vi "writeToXMLAzimuth.vi"(8 "error in (no error)":errorcluster, 10 "Class Label":string="Azimuth") -> (0 "error out":errorcluster, 2 "XML out":string="<Azimuth>\n  <degreesArc>0</degreesArc>\n  <minutesArc>0</minutesArc>\n  <secondsArc>0</secondsArc>\n</Azimuth>")   [LabVIEW 2012]
uses:
  <userlib>/Common/UnitsAndXML/FlattenItemWithUnitToXML/FlattenPlaneAngleToXML/PlaneAngleUnit.ctl
  <userlib>/Common/UnitsAndXML/UnitsAndXML.lvlib
panel:
  in  "degreesAlt":dbl[unit]=0.7330382858376184
  in  "secondsArc":dbl[unit]=0.0002617993877991494
  in  "minutesArc":dbl[unit]=0.00930842267730309
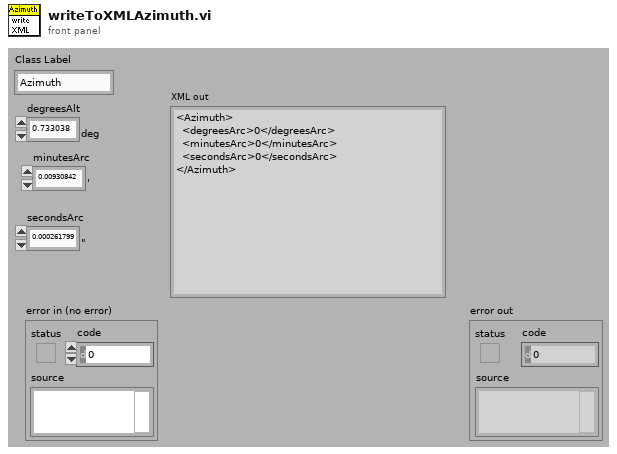
[diagram p1: front panel]
types:
  T1 = typedef "UnitsAndXML.lvlib/PlaneAngleUnit.ctl" = enum16{"rad", "deg", "'", "\""}
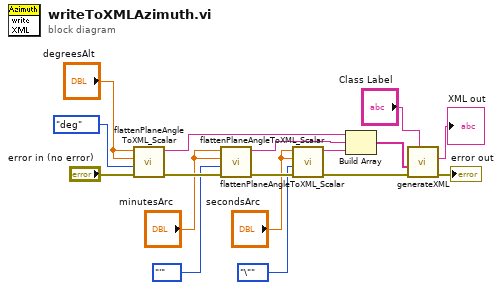
[diagram p0: block diagram]
diagram:
  n1 = call <userlib>:"flattenPlaneAngleToXML_Scalar.vi"("error in (no error)"="error in (no error)", "planeAngleUnitInXML"=PlaneAngleUnit."deg", "planeAngleAgain"="degreesAlt", "planeAngle"="degreesAlt") -> ("error out"=w14:errorcluster, "xmlString"=w11:string)  [unwired: 6 in]
  n2 = call <userlib>:"flattenPlaneAngleToXML_Scalar.vi"("error in (no error)"=w14, "planeAngleUnitInXML"=PlaneAngleUnit."'", "planeAngleAgain"="minutesArc", "planeAngle"="minutesArc") -> ("error out"=w16:errorcluster, "xmlString"=w10:string)  [unwired: 6 in]
  n3 = call <userlib>:"flattenPlaneAngleToXML_Scalar.vi"("error in (no error)"=w16, "planeAngleUnitInXML"=PlaneAngleUnit."\"", "planeAngleAgain"="secondsArc", "planeAngle"="secondsArc") -> ("error out"=w2:errorcluster, "xmlString"=w9:string)  [unwired: 6 in]
  n4 = Build Array(w11, w10, w9) -> (w4:string[])
  n5 = call <userlib>:"generateXML.vi"("elementName"="Class Label", "error in"=w2, "childrenXML"=w4) -> ("error out"=→"error out":errorcluster, "XML out"=→"XML out":string)  [unwired: 6 in, 1 out]
